vi "Search in DB.vi"(8 "error in (no error)":errorcluster, 11 "DB Data in":T1={"Account"=0, "First Name"="", "Last Name"="", "Balance"=0.0, "DB Info"=enum."Login Accepted"} {"Balance" format="%.2f"; "Account" format="%05d"}) -> (0 "error out":errorcluster, 2 "DB Record":T3 {"Balance" format="%.2f"; "Account" format="%05d"}, 3 "refnum out":refnum<file>)   [LabVIEW 2017]
uses:
  Type Definitions/DB Record.ctl
  Type Definitions/DB Data.ctl
  Type Definitions/DB Info.ctl
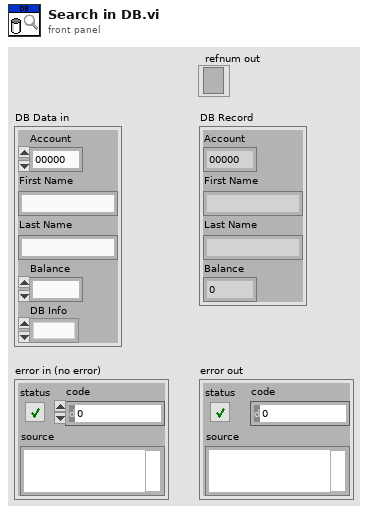
[diagram p1: front panel]
types:
  T1 = typedef "DB Data.ctl" = cluster{"Account":i32, "First Name":string, "Last Name":string, "Balance":fxp<+/-,64,35>, "DB Info":T2}
  T2 = typedef "DB Info.ctl" = enum16{"Empty", "Verify", "Login Accepted", "Invalid Login", "Deposit Complete", "Withdrawal Complete", "Withdrawal Failed", "Terminate"}
  T3 = typedef "DB Record.ctl" = cluster{"Account":i32, "First Name":string, "Last Name":string, "Balance":fxp<+/-,64,35>}
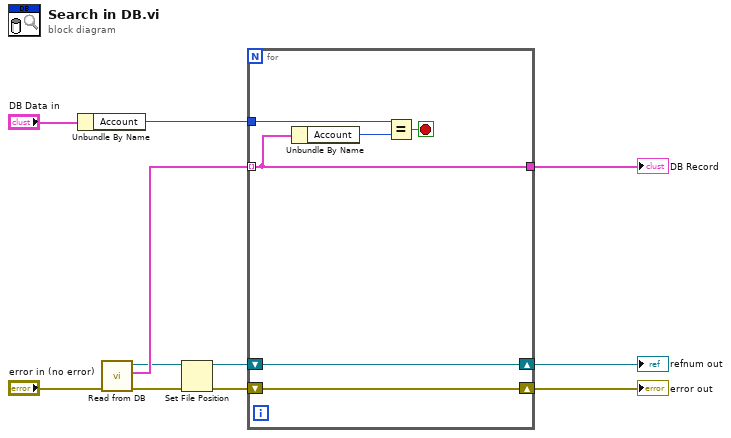
[diagram p0: block diagram]
diagram:
  n1 = Unbundle By Name("DB Data in") -> ("Account"=w9:i32)
  n2 = call "Read from DB.vi"("error in (no error)"="error in (no error)") -> ("error out"=w3:errorcluster, "Array"=w7:T3[], "refnum out"=w4:refnum<file>)  [unwired: 8 in]
  n3 = Set File Position(refnum=w4, error in=w3) -> (refnum out=w1:refnum<file>, error out=w2:errorcluster)  [unwired: 2 in]
  n4 = for {
    tunnel: w7 -> [w13] mode=indexing
    tunnel: w9 -> [w17]
    tunnel: [w13] -> w8
    shift-right: [w14] -> w6
    shift-left: w2 -> [w14]
    shift-right: [w12] -> w5
    shift-left: w1 -> [w12]
    stop <- w15 stop-if-true
    n5 = Unbundle By Name(w13) -> ("Account"=w16:i32)
    n6 = Equal?(x=w17, y=w16) -> (x = y?=w15:bool)
  }
  "DB Record" <- w8
  "error out" <- w6
  "refnum out" <- w5
